vi "Instr_SetPrivateData.vi"(8 "error in (no error)":errorcluster, 11 "KE487 in":refnum<class "KE487.lvclass">) -> (0 "error out":errorcluster, 3 "KE487 out":refnum<class "KE487.lvclass">)   [LabVIEW 2013, in "KE487.lvclass"]
uses:
  KE487.lvclass
  InstrumentSetup.vi
  KE487_CommandsGlobal.vi
  InstrControl.lvclass
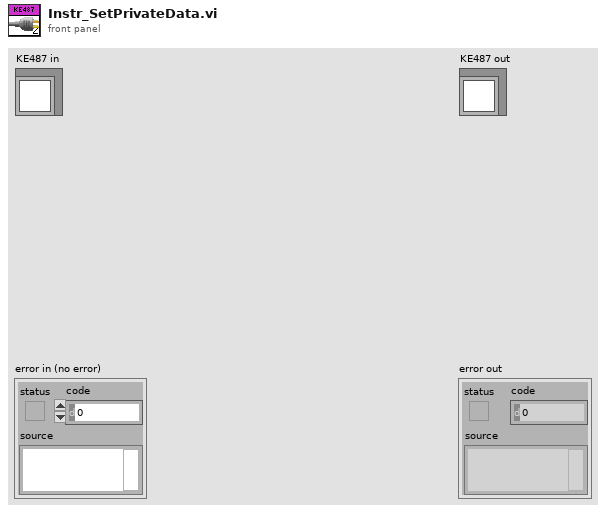
[diagram p1: front panel]
types:
  T1 = cluster{"Compliance":u16, "Range:":u16, "GPIB Address":string}
  T2 = cluster{"GPIB address":string, "Instrument name":string, "Instrument type":u16, "Command \"Reset\"":string, "Command \"Initialise\"":string, "Command \"Arm\"":string, "Command \"SetVolts\"":string, "Command \"Compliance?\"":string, "Command \"Standby\"":string, "Command \"Read Current\"":string}
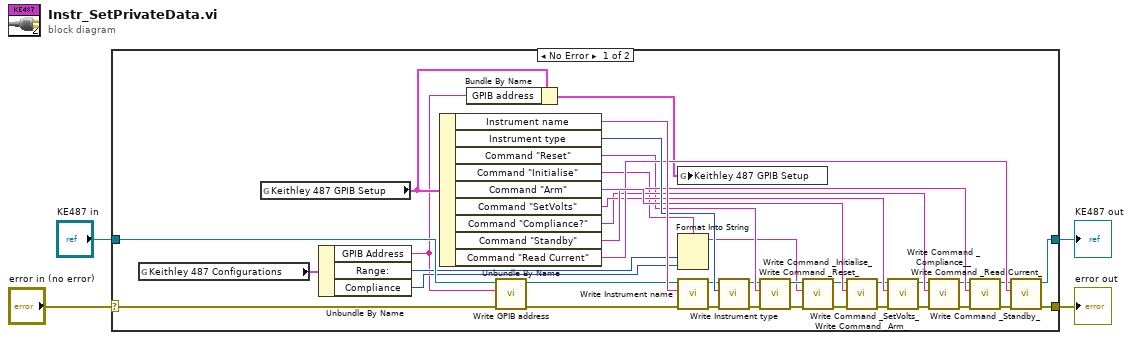
[diagram p0: block diagram]
diagram:
  n1 = case shown="No Error" "error in (no error)" {
    selector: "error in (no error)" -> [w25 w44]
    tunnel: [w14 w44] -> w1
    tunnel: [w15 w43] -> w2
    tunnel: "KE487 in" -> [w13 w43]
    frame No Error {
      n2 = global read "InstrumentSetup.vi" "Keithley 487 Configurations"() -> (w12:T1)
      n3 = global read "KE487_CommandsGlobal.vi" "Keithley 487 GPIB Setup"() -> (w6:T2)
      n4 = Unbundle By Name(w12) -> ("GPIB Address"=w5:string, "Range:"=w11:u16, "Compliance"=w8:u16)
      n5 = Unbundle By Name(w6) -> ("Instrument name"=w42:string, "Instrument type"=w41:u16, "Command \"Reset\""=w35:string, "Command \"Initialise\""=w10:string, "Command \"Arm\""=w40:string, "Command \"SetVolts\""=w37:string, "Command \"Compliance?\""=w36:string, "Command \"Standby\""=w38:string, "Command \"Read Current\""=w39:string)
      n6 = Bundle By Name(cluster=w6, "GPIB address"=w5) -> (w7:T2)
      n7 = call-dynamic "Write GPIB address.vi"("error in (no error)"=w25, "GPIB address"=w5, "InstControl in"=w13) -> ("error out"=w24:errorcluster, "InstControl out"=w34:refnum<class "KE487.lvclass">)  [unwired: 7 in]
      n8 = global write "KE487_CommandsGlobal.vi" "Keithley 487 GPIB Setup"(w7) -> ()
      n9 = Format Into String(format string=w10, w11, w8) -> (resulting string=w9:string)  [unwired: 2 in, 1 out]
      n10 = call-dynamic "Write Instrument name.vi"("error in (no error)"=w24, "Instrument name"=w42, "InstControl in"=w34) -> ("error out"=w23:errorcluster, "InstControl out"=w33:refnum<class "KE487.lvclass">)  [unwired: 7 in]
      n11 = call-dynamic "Write Instrument type.vi"("error in (no error)"=w23, "Instrument type"=w41, "InstControl in"=w33) -> ("error out"=w22:errorcluster, "InstControl out"=w32:refnum<class "KE487.lvclass">)  [unwired: 7 in]
      n12 = call-dynamic "Write Command _Reset_.vi"("error in (no error)"=w22, "Command \"Reset\""=w35, "SupplyControl in"=w32) -> ("error out"=w21:errorcluster, "SupplyControl out"=w31:refnum<class "KE487.lvclass">)  [unwired: 7 in]
      n13 = call-dynamic "Write Command _Initialise_.vi"("error in (no error)"=w21, "Command \"Initialise\""=w9, "SupplyControl in"=w31) -> ("error out"=w20:errorcluster, "SupplyControl out"=w30:refnum<class "KE487.lvclass">)  [unwired: 7 in]
      n14 = call-dynamic "Write Command _Arm_.vi"("error in (no error)"=w20, "Command \"Arm\""=w40, "SupplyControl in"=w30) -> ("error out"=w19:errorcluster, "SupplyControl out"=w29:refnum<class "KE487.lvclass">)  [unwired: 7 in]
      n15 = call-dynamic "Write Command _SetVolts_.vi"("error in (no error)"=w19, "Command \"SetVolts\""=w37, "SupplyControl in"=w29) -> ("error out"=w18:errorcluster, "SupplyControl out"=w28:refnum<class "KE487.lvclass">)  [unwired: 7 in]
      n16 = call-dynamic "Write Command _Compliance__.vi"("error in (no error)"=w18, "Command \"Compliance?\""=w36, "SupplyControl in"=w28) -> ("error out"=w17:errorcluster, "SupplyControl out"=w27:refnum<class "KE487.lvclass">)  [unwired: 7 in]
      n17 = call-dynamic "Write Command _Standby_.vi"("error in (no error)"=w17, "Command \"Standby\""=w38, "SupplyControl in"=w27) -> ("error out"=w16:errorcluster, "SupplyControl out"=w26:refnum<class "KE487.lvclass">)  [unwired: 7 in]
      n18 = call-dynamic "Write Command _Read Current_.vi"("error in (no error)"=w16, "Command \"Read Current\""=w39, "SupplyControl in"=w26) -> ("error out"=w14:errorcluster, "SupplyControl out"=w15:refnum<class "KE487.lvclass">)  [unwired: 7 in]
    }
    frame Error {
    }
  }
  "error out" <- w1
  "KE487 out" <- w2
